vi "Declare Dependency.vi"(6 "Shared Resource (F)":bool, 7 "Dependency":refnum<class "Dependency.lvclass">, 8 "error in (no error)":errorcluster, 9 "Start Order (0)":i8, 10 "Name":string, 11 "Type":refnum<class "SMO.lvclass">) -> (0 "error out":errorcluster, 3 "Dependency out":refnum<class "Dependency.lvclass">)   [LabVIEW 2013, in "Dependency.lvclass"]
uses:
  Dependency.lvclass
  SMO/SMO.lvclass
  Dependency.lvclass/Dependency.ctl
  <vilib>/regexp/Match Regular Expression.xnode
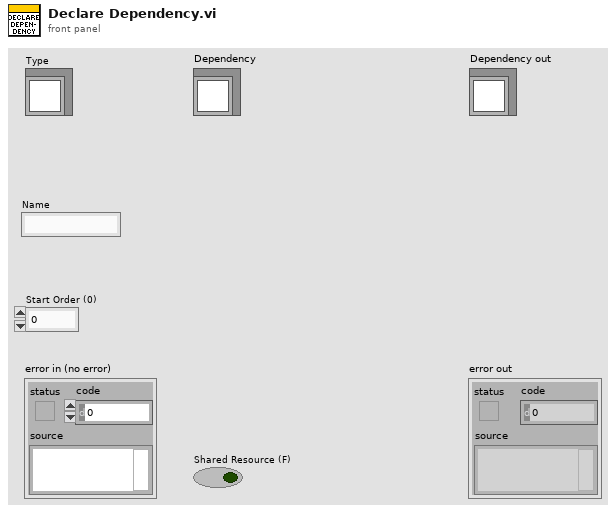
[diagram p1: front panel]
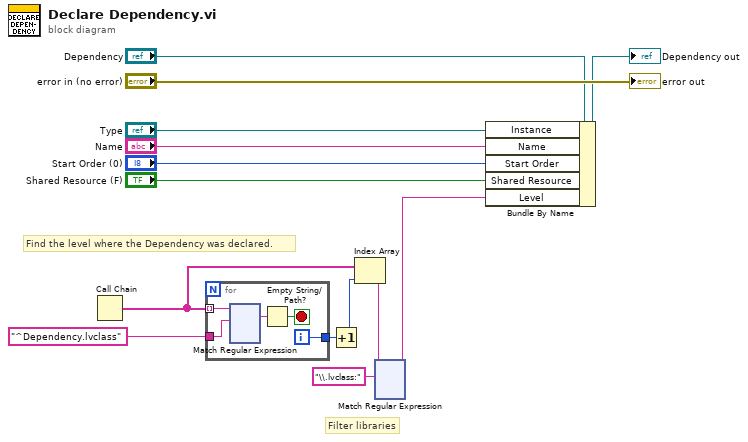
[diagram p0: block diagram]
diagram:
  # "Filter libraries"
  # "Find the level where the Dependency was declared."
  n1 = Call Chain() -> (call chain=w5:string[])
  n2 = for {
    tunnel: w5 -> [w18] mode=indexing
    tunnel: "^Dependency.lvclass" -> [w17]
    tunnel: [w14] -> w1
    i -> [w14]
    stop <- w15 stop-if-true
    n3 = xnode "Match Regular Expression"("input string"=w18, "regular expression"=w17) -> ("whole match"=w16:string)  [unwired: 4 in, 4 out]
    n4 = Empty String/Path?(string/path=w16) -> (empty?=w15:bool)
  }
  n5 = Increment(x=w1) -> ()  [unwired: 1 out]
  n6 = Index Array(array=w5, index=w1) -> (element=w4:string)
  n7 = xnode "Match Regular Expression"("input string"=w4, "regular expression"="\\.lvclass:") -> ("before match"=w2:string)  [unwired: 4 in, 4 out]
  n8 = Bundle By Name(cluster="Dependency", "Instance"="Type", "Name"="Name", "Start Order"="Start Order (0)", "Shared Resource"="Shared Resource (F)", "Level"=w2) -> (→"Dependency out":refnum<class "Dependency.lvclass">)
  "error out" <- "error in (no error)"
